vi "Send Message to Current Process.vi"(0 "message queue in":T1, 5 "message":T2, 9 "timeout (-1 ms)":i32=-1, 11 "error in":errorcluster) -> (4 "message queue out":T1, 10 "timed out?":bool, 15 "error out":errorcluster)   [LabVIEW 2015, in "Car Wash.lvlib" / "AMC.lvlib"]
uses:
  AMC.lvlib
  Tools/Keyed Array/KeyedArray.ctl
  Tools/Keyed Array/Tools_KeyedArray.lvlib
  Message.ctl
  Message Queue.ctl
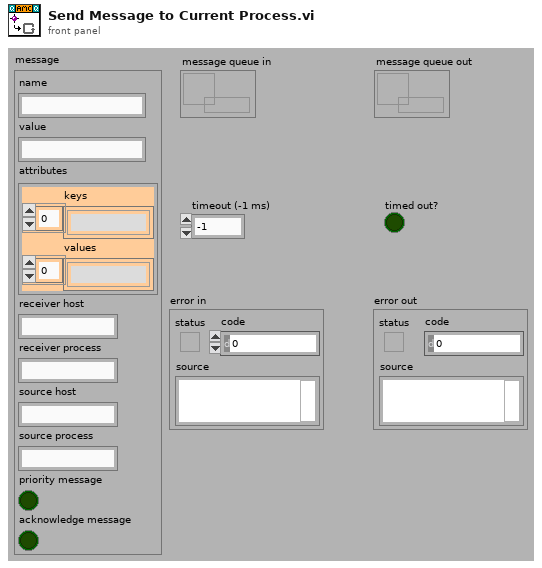
[diagram p1: front panel]
types:
  T1 = typedef "Car Wash.lvlib/AMC.lvlib/Message Queue.ctl" = refnum<queue>
  T2 = typedef "Car Wash.lvlib/AMC.lvlib/Message.ctl" = cluster{"name":string, "value":string, "attributes":T3, "receiver host":string, "receiver process":string, "source host":string, "source process":string, "priority message":bool, "acknowledge message":bool}
  T3 = typedef "Car Wash.lvlib/Tools_KeyedArray.lvlib/KeyedArray.ctl" = cluster{"keys":string[], "values":string[]}
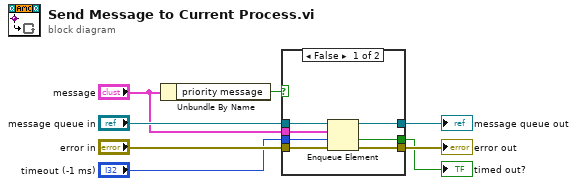
[diagram p0: block diagram]
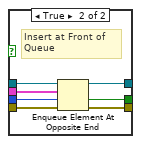
[diagram p2: hidden frame]
diagram:
  n1 = Unbundle By Name("message") -> ("priority message"=w1:bool)
  n2 = case shown="False" w1 {
    tunnel: "message queue in" -> [w15 w19]
    tunnel: [w14 w20] -> w8
    tunnel: [w13 w21] -> w6
    tunnel: "error in" -> [w12 w22]
    tunnel: "message" -> [w11 w18]
    tunnel: "timeout (-1 ms)" -> [w10 w17]
    tunnel: [w9 w16] -> w3
    frame False {
      n3 = Enqueue Element(queue=w15, element=w11, timeout in ms (-1)=w10, error in (no error)=w12) -> (queue out=w14:T1, timed out?=w9:bool, error out=w13:errorcluster)
    }
    frame True {
      # "Insert at Front of Queue"
      n4 = Enqueue Element At Opposite End(queue=w19, element=w18, timeout in ms (-1)=w17, error in (no error)=w22) -> (queue out=w20:T1, timed out?=w16:bool, error out=w21:errorcluster)
    }
  }
  "message queue out" <- w8
  "error out" <- w6
  "timed out?" <- w3
